vi "Try Parse.vi"(0 "SG Path in":refnum<class "SG 18GHz Path.lvclass">, 5 "Config Row":string[](array[string]), 11 "error in":errorcluster) -> (4 "SG Path out":refnum<class "SG 18GHz Path.lvclass">, 6 "Is of type?":bool=TRUE, 15 "error out":errorcluster)   [LabVIEW 2023, in "RFFixtureCharact.RFPM.lvlib" / "SG 18GHz Path.lvclass"]
uses:
  SG 18GHz Path.lvclass
  Common/RFCalAndFixtureCharact.Common.lvlib
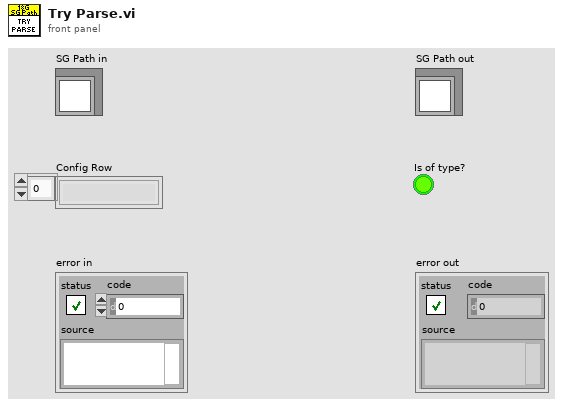
[diagram p1: front panel]
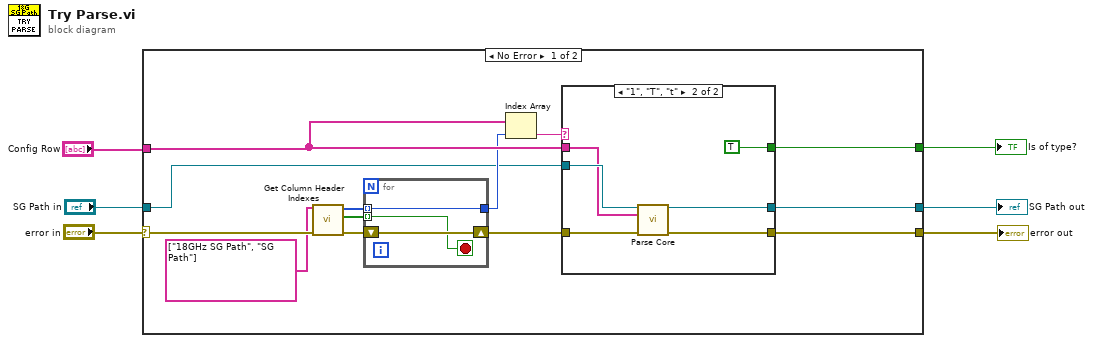
[diagram p0: block diagram]
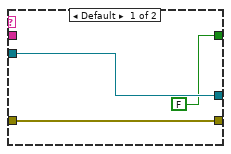
[diagram p2: hidden frame]
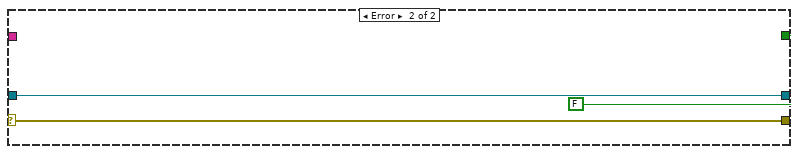
[diagram p3: hidden frame]
diagram:
  n1 = case shown="No Error" "error in" {
    selector: "error in" -> [w18 w34]
    tunnel: [w11 w34] -> w3
    tunnel: [w19 FALSE ("Is of type?")] -> w2
    tunnel: [w10 w33] -> w1
    tunnel: "Config Row" -> [w17 _]
    tunnel: "SG Path in" -> [w12 w33]
    frame No Error {
      n2 = call "Get Column Header Indexes.vi"("Column Header Names"=string[] ["18GHz SG Path", "SG Path"], "error in"=w18) -> ("Column Header Indices"=w14:i32[], "Column Header Exists?"=w8:bool[], "error out"=w9:errorcluster)  [unwired: 11 in]
      n3 = for {
        tunnel: w14 -> [w20] mode=indexing
        tunnel: [w20] -> w13
        shift-right: [w22] -> w7
        shift-left: w9 -> [w22]
        tunnel: w8 -> [w21] mode=indexing
        stop <- w21 stop-if-true
      }
      n4 = Index Array(array=w17, index=w13) -> (element=w16:string)
      n5 = case shown="\"1\", \"T\", \"t\"" w16 {
        tunnel: [w23 w31] -> w11
        tunnel: [FALSE ("Is of type?") TRUE ("Is of type?")] -> w19
        tunnel: [w25 w30] -> w10
        tunnel: w7 -> [w23 w29]
        tunnel: w12 -> [w25 w28]
        tunnel: w17 -> [_ w27]
        frame Default {
        }
        frame "1", "T", "t" {
          n6 = call-dynamic "Parse Core.vi"("SG Path in"=w28, "Config Row"=w27, "error in"=w29) -> ("SG Path out"=w30:refnum<class "SG 18GHz Path.lvclass">, "error out"=w31:errorcluster)  [unwired: 11 in]
        }
      }
    }
    frame Error {
    }
  }
  "error out" <- w3
  "SG Path out" <- w1
  "Is of type?" <- w2
